vi "Obtain Request Events.vi"(8 "error in":errorcluster, 10 "Create New? (F)":bool) -> (0 "error out":errorcluster, 2 "Scanner Request Events":T1)   [LabVIEW 2024, in "Scanner.lvlib"]
doc: "This VI Obtains/Creates the Requests events that will be used for other modules to communicate with the module that owns this VI. These Requests events will be accessed only via Public API methods for this module.\n\n<b>NOTE</b>: The contents of this VI are automatically generated and modified by the <b>Tools > DQMH Consortium > DQMH</b> utilities. Consider using those utilities instead of making your own modifications to this VI.\n_____\nBased on DQMH Dev Tools: Project Template 7.1.0.1503."
uses:
  Scanner.lvlib
  Request Events--cluster.ctl
  Stop Argument--cluster.ctl
  Show Panel Argument--cluster.ctl
  Hide Panel Argument--cluster.ctl
  Get Module Execution Status Argument--cluster.ctl
  Show Diagram Argument--cluster.ctl
  connect Argument--cluster.ctl
panel:
  # "NOTE: The contents of this VI are automatically generated and modified by the Tools > DQMH Consortium > DQMH utilities. Consider using those utilities instead of making your own modifications to this VI."
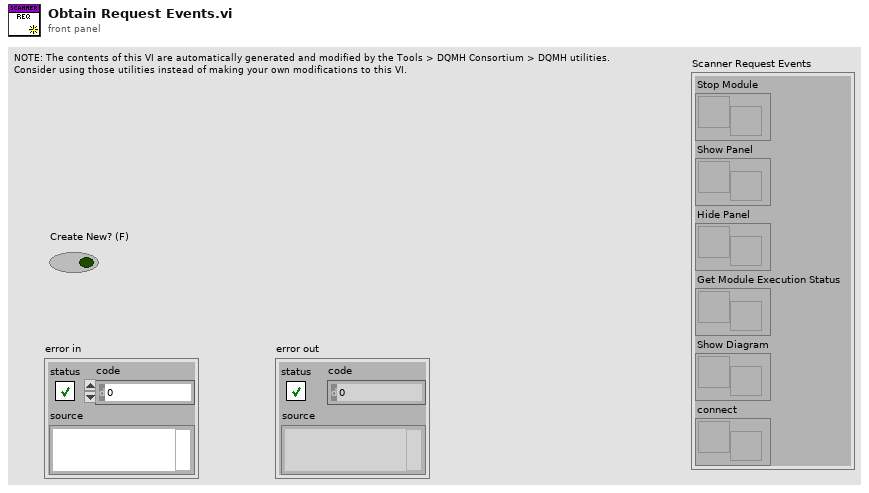
[diagram p1: front panel]
types:
  T1 = typedef "Scanner.lvlib/Request Events--cluster.ctl" = cluster{"Stop Module":refnum<user-event>, "Show Panel":refnum<user-event>, "Hide Panel":refnum<user-event>, "Get Module Execution Status":refnum<user-event>, "Show Diagram":refnum<user-event>, "connect":refnum<user-event>}
  T2 = typedef "Scanner.lvlib/connect Argument--cluster.ctl" = cluster{"VISA":refnum<visa-resource-name>}
  T3 = typedef "Scanner.lvlib/Hide Panel Argument--cluster.ctl" = cluster{"Hide Panel?":bool}
  T4 = typedef "Scanner.lvlib/Show Panel Argument--cluster.ctl" = cluster{"Show Panel?":bool}
  T5 = typedef "Scanner.lvlib/Show Diagram Argument--cluster.ctl" = cluster{"Debug?":bool}
  T6 = typedef "Scanner.lvlib/Get Module Execution Status Argument--cluster.ctl" = cluster{"Running?":bool}
  T7 = typedef "Scanner.lvlib/Stop Argument--cluster.ctl" = cluster{"Origin":string, "Exit via Stop Module Req?":bool, "Wait for Module to stop?":bool}
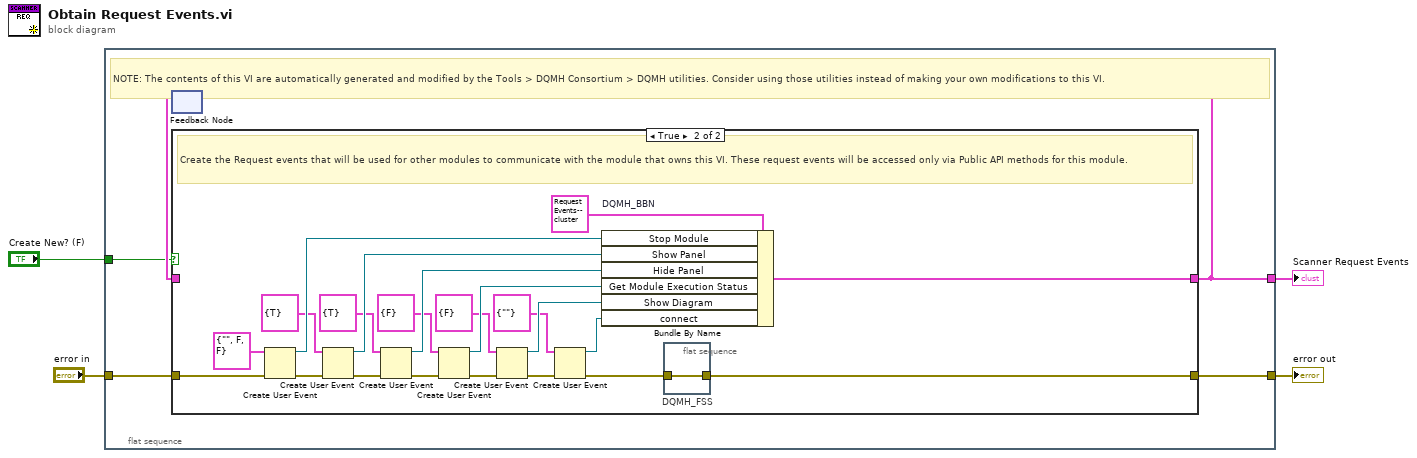
[diagram p0: block diagram]
diagram:
  n1 = flat-sequence {
    tunnel: [w9] -> w4
    tunnel: "error in" -> [w8]
    tunnel: [w6] -> w2
    tunnel: "Create New? (F)" -> [w5]
    frame #0 {
      # "NOTE: The contents of this VI are automatically generated and modified by the Tools > DQMH Consortium > DQMH utilities. Consider using those utilities instead of making your own modifications to this VI."
      n2 = feedback #1() -> (w7:T1)  [unwired: 1 in]
      n3 = case shown="True" w5 {
        tunnel: [w10 w23] -> w9
        tunnel: w8 -> [w10 w33]
        tunnel: [w11 w30] -> w6
        tunnel: w7 -> [w11 _]
        frame False {
          # "Obtain the Request events that were created in a previous call to this VI."
        }
        frame True {
          # "Create the Request events that will be used for other modules to communicate with the module that owns this VI. These request events will be accessed only via Public API methods for this module."
          n4 = Create User Event(user event datatype=T7 {"Origin"="", "Exit via Stop Module Req?"=FALSE, "Wait for Module to stop?"=FALSE} ("Stop Argument"), error in=w33) -> (user event=w31:refnum<user-event>, error out=w28:errorcluster)
          n5 = Create User Event(user event datatype=T4 {"Show Panel?"=TRUE} ("Show Panel Argument"), error in=w28) -> (user event=w27:refnum<user-event>, error out=w26:errorcluster)
          n6 = Create User Event(user event datatype=T3 {"Hide Panel?"=TRUE} ("Hide Panel Argument"), error in=w26) -> (user event=w25:refnum<user-event>, error out=w24:errorcluster)
          n7 = Create User Event(user event datatype=T6 {"Running?"=FALSE} ("Get Module Execution Status Argument"), error in=w24) -> (user event=w21:refnum<user-event>, error out=w22:errorcluster)
          n8 = Create User Event(user event datatype=T5 {"Debug?"=FALSE} ("Show Diagram Argument"), error in=w22) -> (user event=w18:refnum<user-event>, error out=w19:errorcluster)
          n9 = Create User Event(user event datatype=T2 {"VISA"=""} ("connect Argument"), error in=w19) -> (user event=w13:refnum<user-event>, error out=w14:errorcluster)
          n10 = Bundle By Name "DQMH_BBN"(cluster=T1 {"Stop Module"=refnum, "Show Panel"=refnum, "Hide Panel"=refnum, "Get Module Execution Status"=refnum, "Show Diagram"=refnum, "connect"=refnum} ("output cluster"), "Stop Module"=w31, "Show Panel"=w27, "Hide Panel"=w25, "Get Module Execution Status"=w21, "Show Diagram"=w18, "connect"=w13) -> (w30:T1)
          n11 = flat-sequence "DQMH_FSS" {
            tunnel: w14 -> [w34]
            tunnel: [w34] -> w23
            frame #0 {
            }
          }
        }
      }
      n12 = feedback-in #1(w6) -> ()
    }
  }
  "Scanner Request Events" <- w2
  "error out" <- w4
